vi "DB Tools Open Connec (Path).vi"(4 "password":string, 5 "userID":string, 6 "error in (no error)":errorcluster, 7 "connection timeout (15)":i32=15, 8 "prompt? (F)":bool, 9 "connection information":path) -> (0 "error out":errorcluster, 3 "connection reference":T1)   [LabVIEW 2017, in "NI_Database_API.lvlib"]
doc: "Opens a database connection using the connection information path and returns a connection reference. If <B>prompt?</B> is set to TRUE, LabVIEW displays a dialog box to set up the connection. Wire data to the <B>connection information</B> input to determine the polymorphic instance to use or manually select the instance."
uses:
  <vilib>/addons/database/NI_Database_API.lvlib
  <vilib>/addons/database/Connection.llb/Conn ObjectReference.ctl
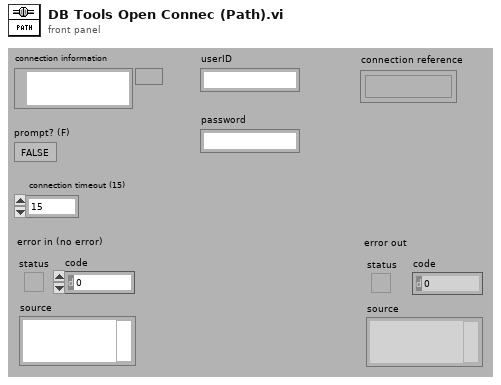
[diagram p1: front panel]
types:
  T1 = typedef "NI_Database_API.lvlib/Conn ObjectReference.ctl" = refnum<k1>
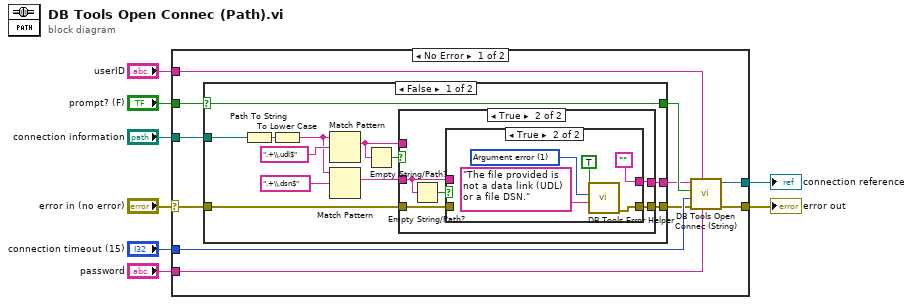
[diagram p0: block diagram]
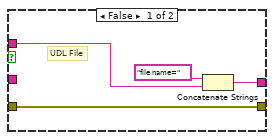
[diagram p2: hidden frame]
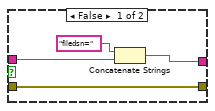
[diagram p3: hidden frame]
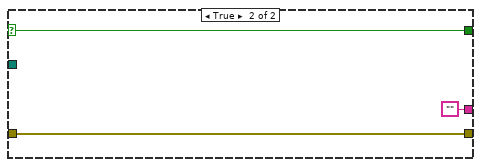
[diagram p4: hidden frame]
diagram:
  n1 = case shown="No Error" "error in (no error)" {
    selector: "error in (no error)" -> [w10 w53]
    tunnel: "prompt? (F)" -> [w19 _]
    tunnel: "connection timeout (15)" -> [w16 _]
    tunnel: "userID" -> [w15 _]
    tunnel: "password" -> [w14 _]
    tunnel: [w13 _] -> w4
    tunnel: [w12 w53] -> w3
    tunnel: "connection information" -> [w9 _]
    frame No Error {
      n2 = case shown="False" w19 {
        selector: w19 -> [w31 w52]
        tunnel: [w31 w52] -> w18
        tunnel: [w23 ""] -> w17
        tunnel: w10 -> [w22 w50]
        tunnel: [w21 w50] -> w11
        tunnel: w9 -> [w20 _]
        frame False {
          n3 = Path To String(path=w20) -> (string=w30:string)
          n4 = To Lower Case(string=w30) -> (all lower case string=w27:string)
          n5 = Match Pattern(string=w27, regular expression=".+\\.udl$") -> (match substring=w25:string)  [unwired: 4 out]
          n6 = Match Pattern(string=w27, regular expression=".+\\.dsn$") -> (match substring=w24:string)  [unwired: 4 out]
          n7 = Empty String/Path?(string/path=w25) -> (empty?=w26:bool)
          n8 = case shown="True" w26 {
            tunnel: w25 -> [w35 _]
            tunnel: [w33 w40] -> w23
            tunnel: w24 -> [_ w39]
            tunnel: w22 -> [w32 w37]
            tunnel: [w32 w36] -> w21
            frame False {
              # "UDL File"
              n9 = Concatenate Strings("file name=" ("Substring"), w35) -> (w33:string)
            }
            frame True {
              n10 = Empty String/Path?(string/path=w39) -> (empty?=w38:bool)
              n11 = case shown="True" w38 {
                tunnel: w39 -> [w43 _]
                tunnel: [w42 ""] -> w40
                tunnel: [w41 w48] -> w36
                tunnel: w37 -> [w41 _]
                frame False {
                  n12 = Concatenate Strings("filedsn=" ("Substring"), w43) -> (w42:string)
                }
                frame True {
                  w47 = 1 items=["No error", "Argument error", "Memory is full", "Out of zone", "End of file", "File already open", "Generic file I/O error", "File not found", "File permission error", "Disk is full", "Duplicate path", "Too many files open", "System feature not enabled", "Resource file not found", "Cannot add resource", "Resource not found", "Image not found", "Image memory error", "Pen does not exist", "Config type invalid", "Config token not found", "Config parse error", "Config memory error", "Bad external code format", "Bad external code offset", "External code not present", "Null window", "Destroy window error", "Null menu", "Print aborted", "Bad print record", "Print driver error", "Windows error during printing", "Memory error during printing", "Print dialog error", "Generic print error", "Invalid device refnum", "Device not found", "Device parameter error", "Device unit error", "Cannot open device", "Device call aborted", "Generic error", "Cancelled by user", "Object ID too low", "Object ID too high", "Object not in heap", "Unknown heap", "Unknown object (invalid DefProc)", "Unknown object (DefProc not in table)", "Message out of range", "Invalid (null) method", "Unknown message", "Manager call not supported", "Bad address", "Network operation in progress", "Network operation timed out", "Connection is busy", "Network attribute not supported", "Network error", "Address in use", "System out of memory", "Connection aborted", "Connection refused", "Not connected", "Already connected", "Connection closed", "Initialization error (interapplication manager)", "Bad occurrence", "Wait on unbound occurrence handler", "Occurrence queue overflow", "Datalog type conflict", "Unused", "Unrecognized type (interapplication manager)", "Memory corrupt", "Failed to make temporary DLL", "Old CIN version", "Drag socket not found", "Failed to load drop-object", "Failed to register OLE object", "Failed to release OLE object", "Format specifier type mismatch", "Unknown format specifier", "Too few format specifiers", "Too many format specifiers", "Scan failed", "Newer CIN version", "Error converting to variant", "Runtime menu error", "Password tampered", "Variant attribute not found", "Incompatible variant data type", "Event data is not available", "Event Store is not present", "Occurrence is not found", "Event Queue is not created", "Event info is not available", "Refnum passed is NULL", "Error retrieving Class GUID", "Error retrieving CoClass GUID", "Error retrieving TypeLib GUID.", "Bad built application magic bytes.", "Specific driver is different from the specific driver associated with the Logical Name.", "There is no session opened to the class driver.", "Max Error", "MAX - Error with config objects", "MAX - Error loading configuration", "MAX - Group not supported"]
                  n13 = call <vilib>:"DB Tools Error Helper.vi"("source"="The file provided is not a data link (UDL) or a file DSN.", "code"=w47, "status"=TRUE) -> ("error out"=w48:errorcluster)  [unwired: 1 in, 7 out]
                }
              }
            }
          }
        }
        frame True {
        }
      }
      n14 = call <vilib>:"DB Tools Open Connec (String).vi"("password"=w14, "userID"=w15, "error in (no error)"=w11, "connection timeout (15)"=w16, "prompt? (F)"=w18, "connection information"=w17) -> ("error out"=w12:errorcluster, "connection reference"=w13:T1)  [unwired: 2 out]
    }
    frame Error {
    }
  }
  "error out" <- w3
  "connection reference" <- w4
